vi "Run Step.vi"(0 "CAN Cmd Ref":refnum<vi>, 2 "FPGA Ref":refnum<k20>, 3 "Stagger Time (ms)":i32, 4 "Cycles Completed in":u32, 5 "PWM Freq (Hz)":dbl, 7 "Controller Type:":T3, 8 "# of Steps":i32, 9 "Restarts Cluster":T4={"CMD Starts:"=[0, 0, 0, 0, 0, 0], "Restarts:"=[0, 0, 0, 0, 0, 0], "Total CMD:"=[0, 0, 0, 0, 0, 0], "Total Restarts:"=[0, 0, 0, 0, 0, 0]}, 10 "VoltCtrlRef":string, 13 "Stagger Counter":i32, 14 "Current Step in":i32, 15 "Last CMDs":dbl[](array[numeric]), 16 "Profile":string[][](array[string]), 17 "Pumps Present":u32) -> (12 "PS Cmd":dbl, 18 "Controls":T1, 19 "Ignition Relays":T2, 20 "Manual CMDs":dbl[](array[numeric]), 21 "Current Step out":i32, 23 "Press Cmd":dbl, 24 "Cycles Completed out":u32, 25 "Step Time":dbl, 26 "Power Relays":T2, 27 "Restarts Cluster OUT":T4)   [LabVIEW 2013]
uses:
  Type Defs/Restarts Cluster.ctl
  Type Defs/Controller Names.ctl
  <vilib>/rvi/interface/common/niFpgaWaitOnOcc.vi
  <vilib>/Utility/error.llb/Error Cluster From Error Code.vi
  <vilib>/rvi/errors/niLvFpgaAdjustHostInterfaceError.vi
  <vilib>/rvi/interface/nirviReadWriteControl/nirviReadWriteControl.xnode
  NiFpgaLv.dll
  <vilib>/rvi/interface/Simulation/niFpgaSimulationCallBeginRW.vi
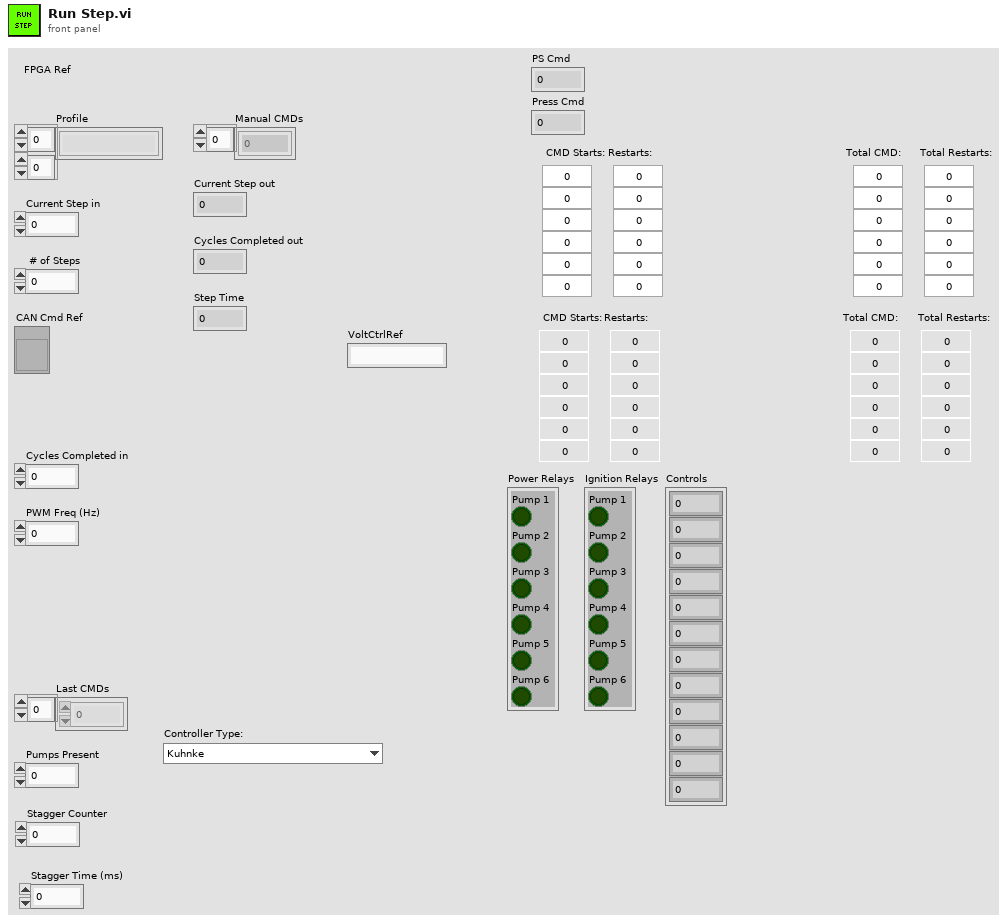
[diagram p1: front panel]
types:
  T1 = cluster{dbl, dbl, dbl, dbl, dbl, dbl, dbl, dbl, dbl, dbl, dbl, dbl}
  T2 = cluster{"Pump 1":bool, "Pump 2":bool, "Pump 3":bool, "Pump 4":bool, "Pump 5":bool, "Pump 6":bool}
  T3 = typedef "Controller Names.ctl" = enum16{"Kuhnke", "Conti", "Helbako", "TI PWM", "PSA", "Hella Gas", "Hella Diesel", "8 Comm", "10 Comm", "8 Comm Hella", "10 Comm Hella", "8 Comm Omron", "10 Comm Omron", "8 Comm Nissan", "10 Comm Nissan"}
  T4 = typedef "Restarts Cluster.ctl" = cluster{"CMD Starts:":i32[], "Restarts:":i32[], "Total CMD:":i32[], "Total Restarts:":i32[]}
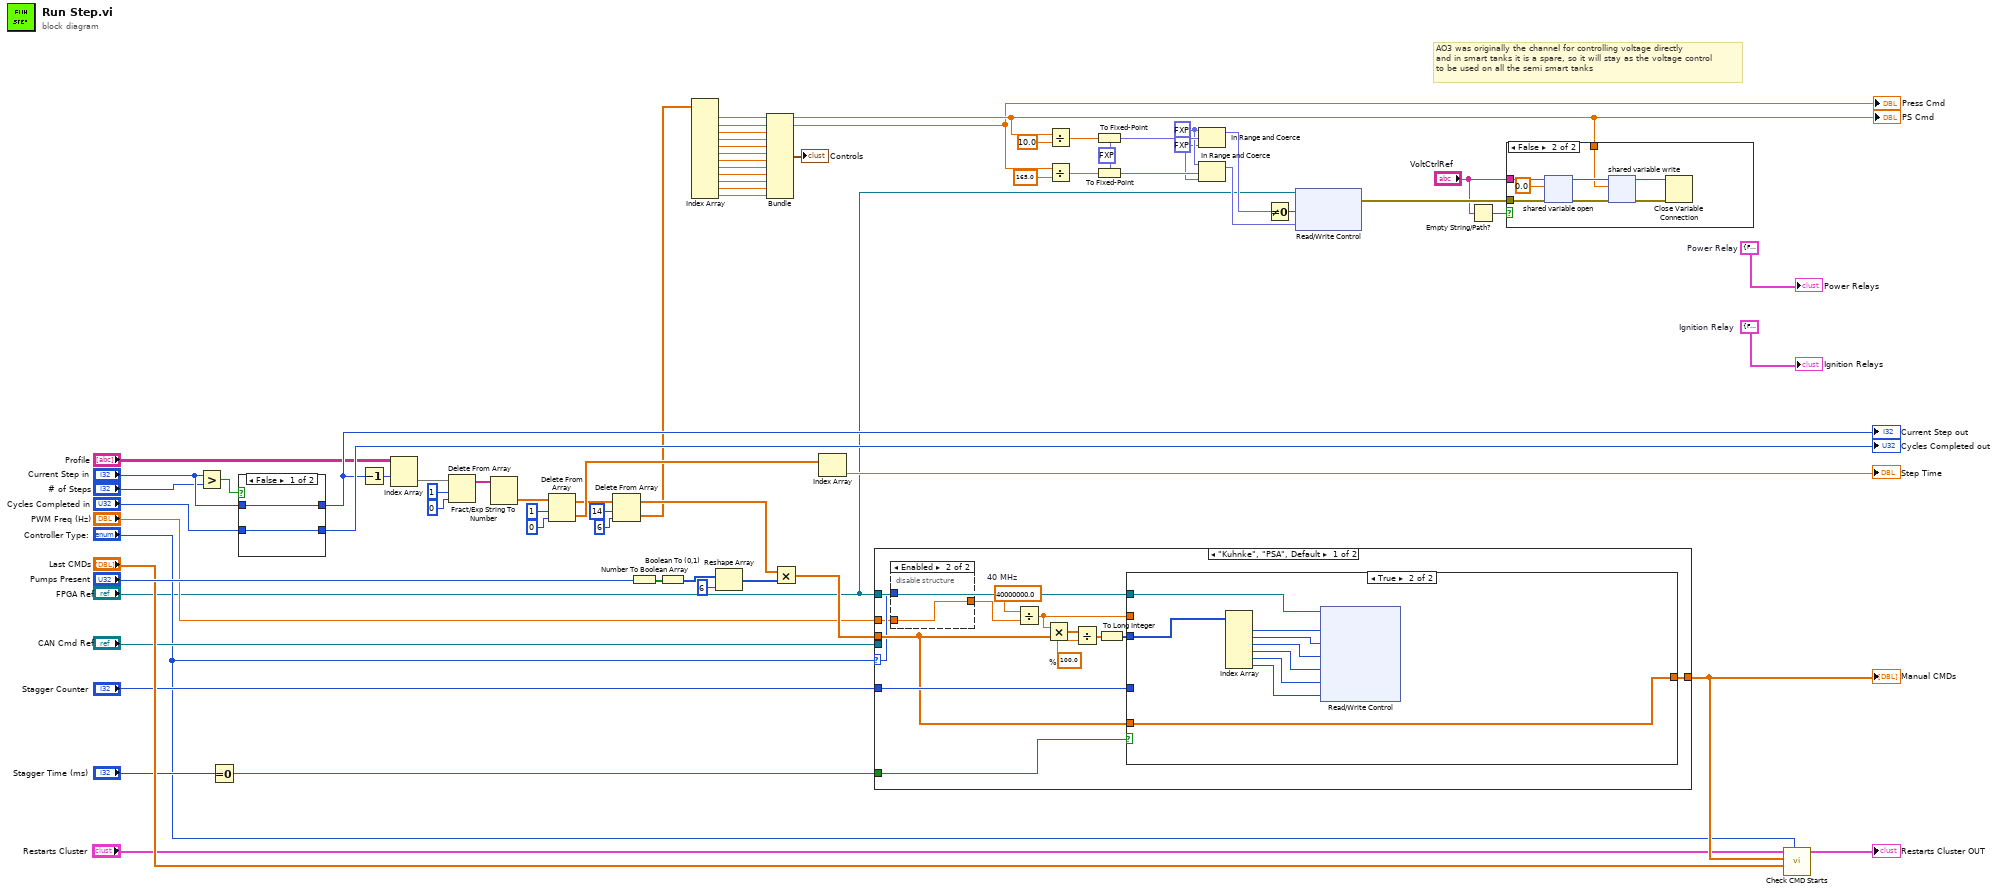
[diagram p0: block diagram]
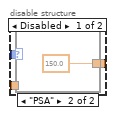
[diagram p3: hidden frame]
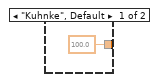
[diagram p4: hidden frame]
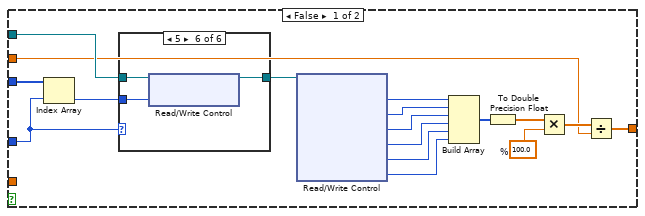
[diagram p5: hidden frame]
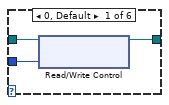
[diagram p6: hidden frame]
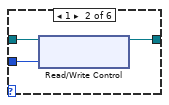
[diagram p7: hidden frame]
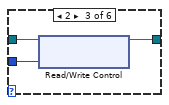
[diagram p8: hidden frame]
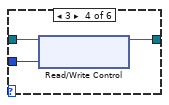
[diagram p9: hidden frame]
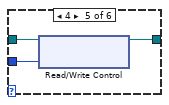
[diagram p10: hidden frame]
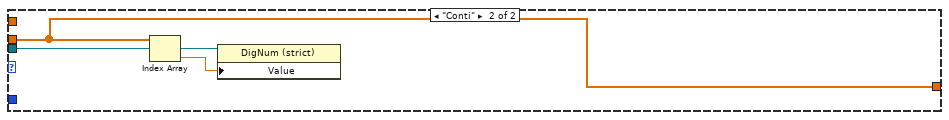
[diagram p11: hidden frame]
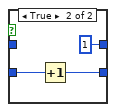
[diagram p12: hidden frame]
diagram:
  w2 = T2 {"Pump 1"=FALSE, "Pump 2"=FALSE, "Pump 3"=FALSE, "Pump 4"=FALSE, "Pump 5"=FALSE, "Pump 6"=FALSE}  # Ignition Relay
  w3 = T2 {"Pump 1"=FALSE, "Pump 2"=FALSE, "Pump 3"=FALSE, "Pump 4"=FALSE, "Pump 5"=FALSE, "Pump 6"=FALSE}  # Power Relay
  w26 = fxp<+/-,20,5> 0.0 ("lower limit")
  w27 = fxp<+/-,20,5> 5.0 ("upper limit")
  w37 = fxp<+/-,20,5> 0.0 ("AO0")
  # "AO3 was originally the channel for controlling voltage directly\nand in smart tanks it is a spare, so it will stay as the voltage control\nto be used on all the semi smart tanks"
  n1 = Greater?(x="Current Step in", y="# of Steps") -> (0:w62:bool)
  n2 = Equal To 0?(x="Stagger Time (ms)") -> (x = 0?=w40:bool)
  n3 = case shown="False" w62 {
    tunnel: [w71 1 ("Current Step")] -> w64
    tunnel: "Current Step in" -> [w71 _]
    tunnel: "Cycles Completed in" -> [w70 w73]
    tunnel: [w70 w72] -> w66
    frame False {
    }
    frame True {
      n4 = Increment(x=w73) -> (x+1=w72:u32)
    }
  }
  "Cycles Completed out" <- w66
  "Current Step out" <- w64
  n5 = Decrement(x=w64) -> (x-1=w50:i32)
  n6 = Index Array(array="Profile", index (row)=w50) -> (element=w51:string[])  [unwired: 1 in]
  n7 = Delete From Array(array=w51, length=1, index=0 ("length")) -> (array with subset deleted=w55:string[])  [unwired: 1 out]
  n8 = Fract/Exp String To Number(string=w55) -> (number=w58:dbl[])  [unwired: 3 in, 1 out]
  n9 = Delete From Array(array=w58, length=1, index=0 ("length")) -> (deleted portion=w59:dbl[], array with subset deleted=w47:dbl[])
  n10 = Delete From Array(array=w47, length=14, index=6) -> (deleted portion=w18:dbl[], array with subset deleted=w44:dbl[])
  n11 = Number To Boolean Array(number="Pumps Present") -> (Boolean array=w36:bool[])
  n12 = Boolean To (0,1)(Boolean=w36) -> (0, 1=w21:i16[])
  n13 = Index Array(array=w18) -> (element #1=w5:dbl, element #2=w4:dbl, element #3=w17:dbl, element #4=w16:dbl, element #5=w15:dbl, element #6=w14:dbl, element #7=w13:dbl, element #8=w12:dbl, element #9=w11:dbl, element #10=w10:dbl, element #11=w9:dbl, element #12=w8:dbl)  [unwired: 12 in]
  "PS Cmd" <- w5
  "Press Cmd" <- w4
  n14 = Reshape Array(w21, 6 ("dimension size")) -> (w20:i16[])
  n15 = Bundle(w5, w4, w17, w16, w15, w14, w13, w12, w11, w10, w9, w8) -> (→"Controls":T1)  [unwired: 1 in]
  n16 = Multiply(x=w44, y=w20) -> (x*y=w69:dbl[])
  n17 = Index Array(array=w59) -> (element=→"Step Time":dbl)  [unwired: 1 in]
  n18 = case shown="\"Kuhnke\", \"PSA\", Default" "Controller Type:" {
    selector: "Controller Type:" -> [w77 _]
    tunnel: "PWM Freq (Hz)" -> [w75 _]
    tunnel: w69 -> [w78 w138]
    tunnel: "FPGA Ref" -> [w83 _]
    tunnel: "CAN Cmd Ref" -> [_ w139]
    tunnel: "Stagger Counter" -> [w82 _]
    tunnel: [w80 w138] -> w42
    tunnel: w40 -> [w79 _]
    frame "Kuhnke", "PSA", Default {
      w87 = 40000000.0  # 40 MHz
      w85 = 100.0  # %
      n19 = disable-structure shown="Enabled" {
        disable-tunnel: w77 -> [w90 _]
        disable-tunnel: [w89 w93] -> w76
        disable-tunnel: w75 -> [_ w93]
        frame Disabled {
          n20 = case shown="\"PSA\"" w90 {
            tunnel: [100.0 ("y") 150.0 ("y")] -> w89
            frame "Kuhnke", Default {
            }
            frame "PSA" {
            }
          }
        }
        frame Enabled {
        }
      }
      n21 = Divide(x=w87, y=w76) -> (x/y=w81:dbl)
      n22 = Multiply(x=w81, y=w78) -> (x*y=w84:dbl[])
      n23 = Divide(x=w84, y=w85) -> (x/y=w86:dbl[])
      n24 = To Long Integer(number=w86) -> (32bit integer=w88:i32[])
      n25 = case shown="True" w79 {
        tunnel: w88 -> [w110 w137]
        tunnel: w83 -> [w109 w129]
        tunnel: w82 -> [w107 _]
        tunnel: w81 -> [w95 _]
        tunnel: [w94 w136] -> w80
        tunnel: w78 -> [_ w136]
        frame False {
          w97 = 100.0  # %
          n26 = Index Array(array=w110, index=w107) -> (element=w108:i32)
          n27 = case shown="5" w107 {
            tunnel: w109 -> [w113 w116 w119 w122 w125 w128]
            tunnel: w108 -> [w112 w115 w118 w121 w124 w127]
            tunnel: [w111 w114 w117 w120 w123 w126] -> w106
            frame 0, Default {
              n28 = xnode "Read/Write Control"("FPGA VI Reference In"=w113, "Duty (Ticks) 1"=w112) -> ("FPGA VI Reference Out"=w111:refnum<k20>)  [unwired: 1 in, 1 out]
            }
            frame 1 {
              n29 = xnode "Read/Write Control"("FPGA VI Reference In"=w116, "Duty (Ticks) 2"=w115) -> ("FPGA VI Reference Out"=w114:refnum<k20>)  [unwired: 1 in, 1 out]
            }
            frame 2 {
              n30 = xnode "Read/Write Control"("FPGA VI Reference In"=w119, "Duty (Ticks) 3"=w118) -> ("FPGA VI Reference Out"=w117:refnum<k20>)  [unwired: 1 in, 1 out]
            }
            frame 3 {
              n31 = xnode "Read/Write Control"("FPGA VI Reference In"=w122, "Duty (Ticks) 4"=w121) -> ("FPGA VI Reference Out"=w120:refnum<k20>)  [unwired: 1 in, 1 out]
            }
            frame 4 {
              n32 = xnode "Read/Write Control"("FPGA VI Reference In"=w125, "Duty (Ticks) 5"=w124) -> ("FPGA VI Reference Out"=w123:refnum<k20>)  [unwired: 1 in, 1 out]
            }
            frame 5 {
              n33 = xnode "Read/Write Control"("FPGA VI Reference In"=w128, "Duty (Ticks) 6"=w127) -> ("FPGA VI Reference Out"=w126:refnum<k20>)  [unwired: 1 in, 1 out]
            }
          }
          n34 = xnode "Read/Write Control"("FPGA VI Reference In"=w106) -> ("Duty (Ticks) 1"=w105:i32, "Duty (Ticks) 2"=w104:i32, "Duty (Ticks) 3"=w103:i32, "Duty (Ticks) 4"=w102:i32, "Duty (Ticks) 5"=w101:i32, "Duty (Ticks) 6"=w100:i32)  [unwired: 1 in, 2 out]
          n35 = Build Array(w105, w104, w103, w102, w101, w100) -> (w99:i32[])
          n36 = To Double Precision Float(number=w99) -> (double precision float=w98:dbl[])
          n37 = Multiply(x=w98, y=w97) -> (x*y=w96:dbl[])
          n38 = Divide(x=w96, y=w95) -> (x/y=w94:dbl[])
        }
        frame True {
          n39 = Index Array(array=w137) -> (element #1=w135:i32, element #2=w134:i32, element #3=w133:i32, element #4=w132:i32, element #5=w131:i32, element #6=w130:i32)  [unwired: 6 in]
          n40 = xnode "Read/Write Control"("FPGA VI Reference In"=w129, "Duty (Ticks) 1"=w135, "Duty (Ticks) 2"=w134, "Duty (Ticks) 3"=w133, "Duty (Ticks) 4"=w132, "Duty (Ticks) 5"=w131, "Duty (Ticks) 6"=w130) -> ()  [unwired: 1 in, 2 out]
        }
      }
    }
    frame "Conti" {
      n41 = Index Array(array=w138) -> (element=w140:dbl)  [unwired: 1 in]
      n42 = property class="DigNum (strict)"(reference=w139, "Value"=w140) -> ()  [unwired: 1 in, 2 out]
    }
  }
  "Manual CMDs" <- w42
  n43 = Divide(x=w5, y=10.0) -> (x/y=w30:dbl)
  n44 = Divide(x=w4, y=165.0) -> (x/y=w31:dbl)
  n45 = To Fixed-Point(fixed-point type=w37, number=w30) -> (fixed-point=w35:fxp<+/-,20,5>)
  n46 = To Fixed-Point(fixed-point type=w37, number=w31) -> (fixed-point=w34:fxp<+/-,20,5>)
  n47 = In Range and Coerce(upper limit=w27, x=w35, lower limit=w26) -> (coerced(x)=w28:fxp<+/-,20,5>)  [unwired: 1 out]
  n48 = In Range and Coerce(upper limit=w27, x=w34, lower limit=w26) -> (coerced(x)=w29:fxp<+/-,20,5>)  [unwired: 1 out]
  n49 = Not Equal To 0?(x=w28) -> (x != 0?=w6:bool)
  n50 = xnode "Read/Write Control"("FPGA VI Reference In"="FPGA Ref", "PS Control"=w6, "AO0"=w29) -> ("error out"=w24:errorcluster)  [unwired: 1 in, 1 out]
  n51 = Empty String/Path?(string/path="VoltCtrlRef") -> (empty?=w25:bool)
  n52 = case shown="False" w25 {
    tunnel: w24 -> [_ w144]
    tunnel: w5 -> [_ w142]
    tunnel: "VoltCtrlRef" -> [_ w141]
    frame True {
    }
    frame False {
      n53 = shared-variable-open(w141, w144, 0.0) -> (w148:refnum<k21>, w145:errorcluster)  [unwired: 1 in]
      n54 = shared-variable-write(w148, w145, w142) -> (w147:refnum<k21>, w146:errorcluster)
      n55 = Close Variable Connection(8:w146, 11:w147) -> ()  [unwired: 1 out]
    }
  }
  n56 = call "Check CMD Starts.vi"("Controller Type:"="Controller Type:", "Last CMDs"="Last CMDs", "Current CMDs"=w42, "Restarts Cluster IN"="Restarts Cluster") -> ("Restarts Cluster OUT"=→"Restarts Cluster OUT":T4)  [unwired: 7 in]
  "Power Relays" <- w3
  "Ignition Relays" <- w2
